vi "compress image to 65k_StateM.vi"(5 "Image":T1, 7 "error in (no error)":errorcluster) -> (0 "Data String":string, 3 "error out":errorcluster)   [LabVIEW 2011]
uses:
  IMAQ Image.ctl
  nivision.dll
panel:
  out "x*y":i32
  out "x/y":dbl(graph)
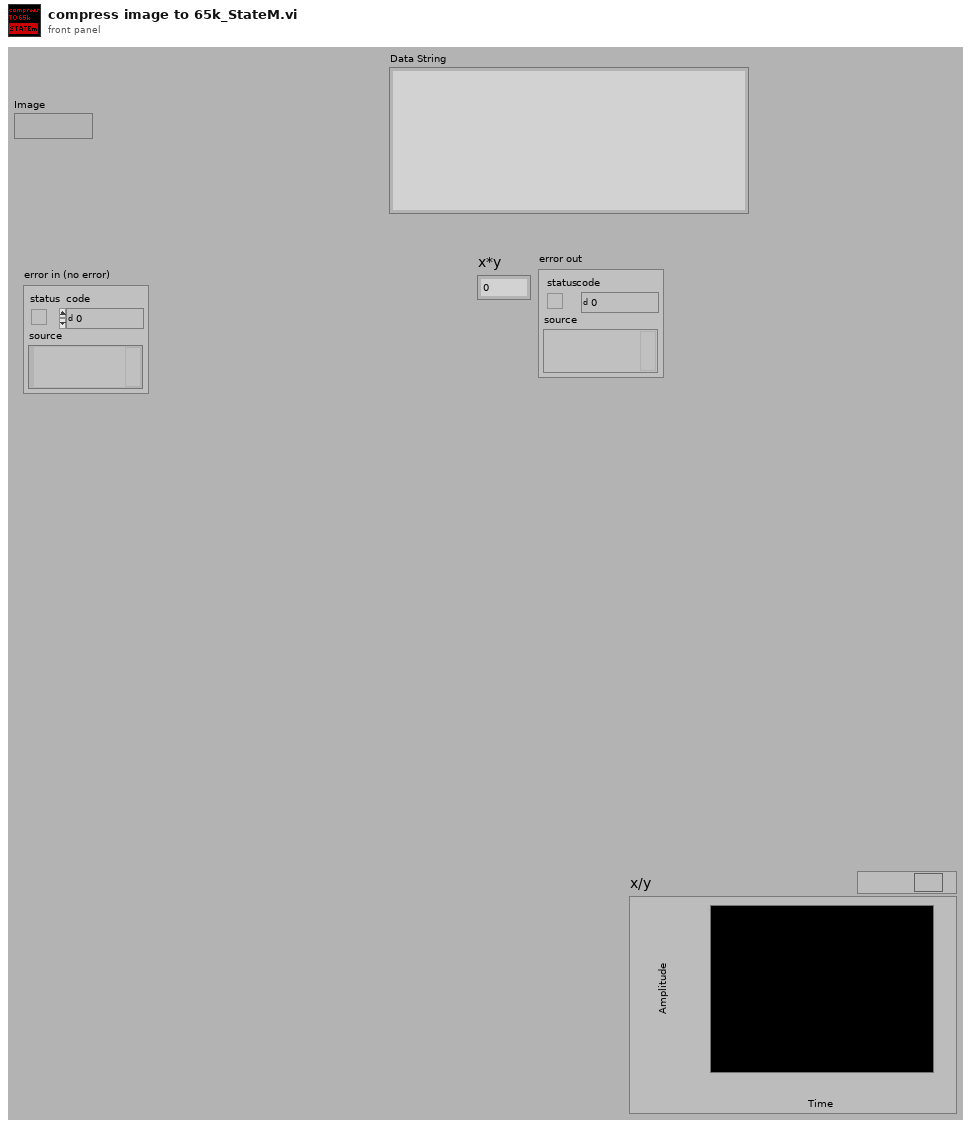
[diagram p1: front panel]
types:
  T1 = typedef "IMAQ Image.ctl" = refnum<image>
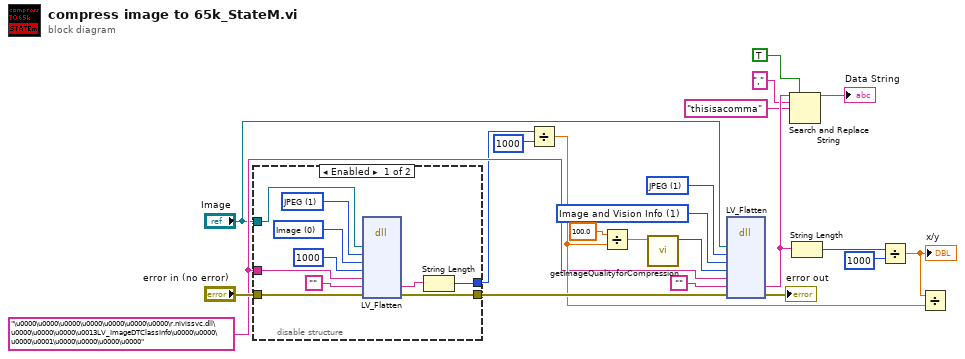
[diagram p0: block diagram]
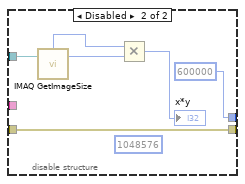
[diagram p2: hidden frame]
diagram:
  w10 = 1 items=["Image", "Image and Vision Info", "Reference to Image"] ("Type of Flatten (Image and Vision Info)")
  w9 = 1 items=["None", "JPEG", "PACKED BINARY"] ("Compression (None)")
  w12 = "\u0000\u0000\u0000\u0000\u0000\u0000\u0000\r.nivissvc.dll\u0000\u0000\u0000\u0013LV_ImageDTClassInfo\u0000\u0000\u0000\u0001\u0000\u0000\u0000\u0000" ("data string")
  n1 = disable-structure shown="Enabled" {
    disable-tunnel: "Image" -> [w32 w37]
    disable-tunnel: "error in (no error)" -> [w31 w38]
    disable-tunnel: [w26 w38] -> w21
    disable-tunnel: w12 -> [w24 _]
    disable-tunnel: [w23 600000 ("Quality (750) 3")] -> w8
    frame Enabled {
      w29 = 0 items=["Image", "Image and Vision Info", "Reference to Image"] ("Type of Flatten (Image and Vision Info)")
      w30 = 1 items=["None", "JPEG", "PACKED BINARY"] ("Compression (None)")
      n2 = dll-call lib="nivision.*" fn="LV_Flatten"("Image"=w32, "compressionType"=w30, "flattenType"=w29, "quality"=1000 ("Quality (750) 3"), "data string"=w24, "output param"="", "error in (no error)"=w31) -> ("output param"=w25:string, "error in (no error)"=w26:errorcluster)  [unwired: 8 in, 3 out]
      n3 = String Length(string=w25) -> (length=w23:i32)
    }
    frame Disabled {
      (unwired) 1048576 ("x*y 2")
      n4 = call "IMAQ GetImageSize"("Image"=w37) -> ("Y Resolution"=w36:i32, "X Resolution"=w35:i32)  [unwired: 3 in, 1 out]
      n5 = Multiply(x=w35, y=w36) -> (x*y=→"x*y":i32)
    }
  }
  n6 = Divide(x=w8, y=1000) -> (x/y=w15:dbl)
  n7 = Divide(x=100.0 ("mean limit in kByte"), y=w15) -> (x/y=w14:dbl)
  n8 = call "getImageQualityforCompression.vi"("compression rate"=w14) -> ("quality"=w13:i16)  [unwired: 10 in]
  n9 = dll-call lib="nivision.*" fn="LV_Flatten"("Image"="Image", "compressionType"=w9, "flattenType"=w10, "quality"=w13, "data string"=w12, "output param"="", "error in (no error)"=w21) -> ("output param"=w5:string, "error in (no error)"=→"error out":errorcluster)  [unwired: 8 in, 3 out]
  n10 = Search and Replace String(replace all?=TRUE ("replace all? (F)"), input string=w5, search string=",", replace string="thisisacomma" ("replace string (\"\")")) -> (result string=→"Data String":string)  [unwired: 4 in, 3 out]
  n11 = String Length(string=w5) -> (length=w20:i32)
  n12 = Divide(x=w20, y=1000) -> (x/y=w17:dbl)
  "x/y" <- w17
  n13 = Divide(x=w17, y=w15) -> ()  [unwired: 1 out]
